vi "Control Mode.vi"(8 "error in (no error)":errorcluster, 10 "Control Mode (1: Remote)":u16(ring)=1 items=["Local", "Remote", "Remote Lock"], 11 "VISA resource name":refnum<visa-resource-name>) -> (0 "error out":errorcluster, 3 "VISA resource name out":refnum<visa-resource-name>)   [LabVIEW 2024, in "Keithley 2200 Series.lvlib"]
doc: "Set the instrument in Local or Remote mode."
uses:
  Keithley 2200 Series.lvlib
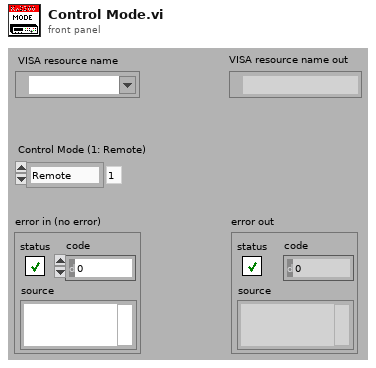
[diagram p1: front panel]
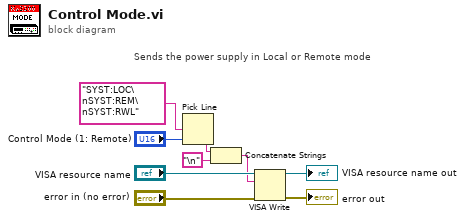
[diagram p0: block diagram]
diagram:
  # "Sends the power supply in Local or Remote mode"
  n1 = Pick Line(multi-line string="SYST:LOC\nSYST:REM\nSYST:RWL", line index="Control Mode (1: Remote)") -> (output string=w5:string)  [unwired: 1 out]
  n2 = Concatenate Strings(w5, "\n") -> (w4:string)
  n3 = VISA Write(VISA resource name="VISA resource name", write buffer=w4, error in (no error)="error in (no error)") -> (VISA resource name out=→"VISA resource name out":refnum<visa-resource-name>, error out=→"error out":errorcluster)  [unwired: 1 out]
